vi "Fit Model to Plot Core.vi"(0 "Fit Plot Information":T6={"XY Graph Ref"=refnum, "Mouse Coordinates"={"X"=0.0, "Y"=0.0}, "Fit Model"=enum."Select a Fit Model...", "Plot Index"=-1}, 1 "LM Function & Gradient":refnum<vi>, 5 "Fit Settings":T3 {"Ramp Type" items=["Linear", "Logarithmic"]; "Fit Method" items=["Least Square", "Least Absolute Residual", "Bisquare"]}, 9 "Additional Data":variant, 11 "error in (no error)":errorcluster, 12 "Bin Location":T2, 13 "Send Graph to Notebook?":bool) -> (3 "Plot Name":string, 4 "Fitted Plot":cluster{"X Array":dbl[], "Y Array":dbl[]}, 6 "Fit Parameters Cluster":variant, 10 "Fit Parameters Uncertainties Cluster":variant, 14 "Fit Algorithm":T1, 15 "error out":errorcluster)   [LabVIEW 2019]
uses:
  Fit Plot Request Information.ctl
  <vilib>/Utility/miscctls.llb/LVPointDoubleTypeDef.ctl
  Fit Models.ctl
  Fit Settings.ctl
  <vilib>/Analysis/6fits.llb/Curve Fitting Criteria.ctl
  Ramp Type.ctl
  Histogram Bin Position.ctl
  Fit Algorithm.ctl
  LabVIEW Plot Interpolation.ctl
  Notebook.lvlib
  <vilib>/Analysis/NI_AALPro.lvlib
panel:
  in  "termination":cluster{"max iteration":i32, "tolerance":dbl}={"max iteration"=2000, "tolerance"=1e-09}
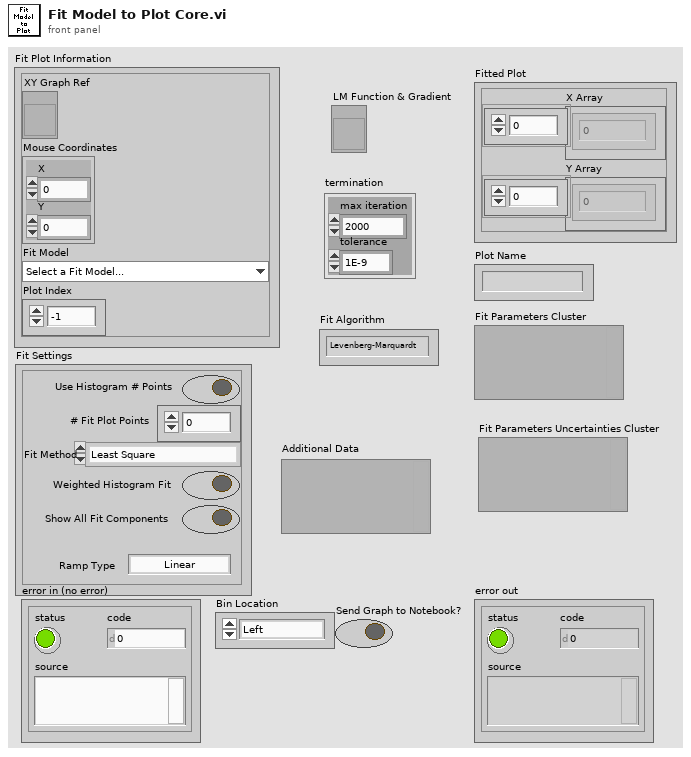
[diagram p1: front panel]
types:
  T1 = typedef "Fit Algorithm.ctl" = enum16{"Levenberg-Marquardt", "Trust-Region Dogleg"}
  T2 = typedef "Histogram Bin Position.ctl" = enum16{"Left", "Center", "Right"}
  T3 = typedef "Fit Settings.ctl" = cluster{"Use Histogram # Points":bool, "# Fit Plot Points":u32, "Fit Method":T4, "Weighted Histogram Fit":bool, "Show All Fit Components":bool, "Ramp Type":T5}
  T4 = typedef "NI_AALPro.lvlib/Curve Fitting Criteria.ctl" = u16
  T5 = typedef "Ramp Type.ctl" = u16
  T6 = typedef "Fit Plot Request Information.ctl" = cluster{"XY Graph Ref":refnum<vi>, "Mouse Coordinates":T7, "Fit Model":T8, "Plot Index":i32}
  T7 = typedef "LVPointDoubleTypeDef.ctl" = cluster{"X":dbl, "Y":dbl}
  T8 = typedef "Fit Models.ctl" = enum16{"Select a Fit Model...", "           Single Peak", "Gaussian", "Asymmetric Gaussian", "Lorentzian", "Asymmetric Lorentzian", "Gaussian/Lorentzian", "Lorentzian/Gaussian", "           Double Peak", "Two Gaussians", "Two Asymmetric Gaussians", "Two H-Connected Gaussians", "Two T-Connected Gaussians", "Two H-Connected Asymmetric Gaussians", "Two T-Connected Asymmetric Gaussians", "           Triple Peak", "Three Gaussians", "Three Asymmetric Gaussians", "              Decays", "Single Exponential", "Two Exponentials", "               ACF", "2D Gaussian ACF", "2D Gaussian + Blinking ACF", "2D Gaussian + Flow ACF", "3D Gaussian ACF", "3D Gaussian + Blinking ACF", "             Multiplot", "2D Gaussian ACF & 2D Gaussian + Flow ACF"}
  T9 = typedef "XY Graph Add-Ons.lvlib/XY Graph Refnum.ctl" = refnum<vi>
  T10 = cluster{"X Array out":dbl[], "Y Array out":dbl[], "Weights":dbl[]}
  T11 = cluster{"parameter minimum":dbl[], "parameter maximum":dbl[]}
  T12 = typedef "Fit Statistics.ctl" = cluster{"# iterations":i32, "number of function calls":i32, "chi2":dbl, "residue":dbl}
  T13 = cluster{"best fit parameters":dbl[], "best nonlinear fit":dbl[]}
  T14 = typedef "LabVIEW Plot Interpolation.ctl" = u8
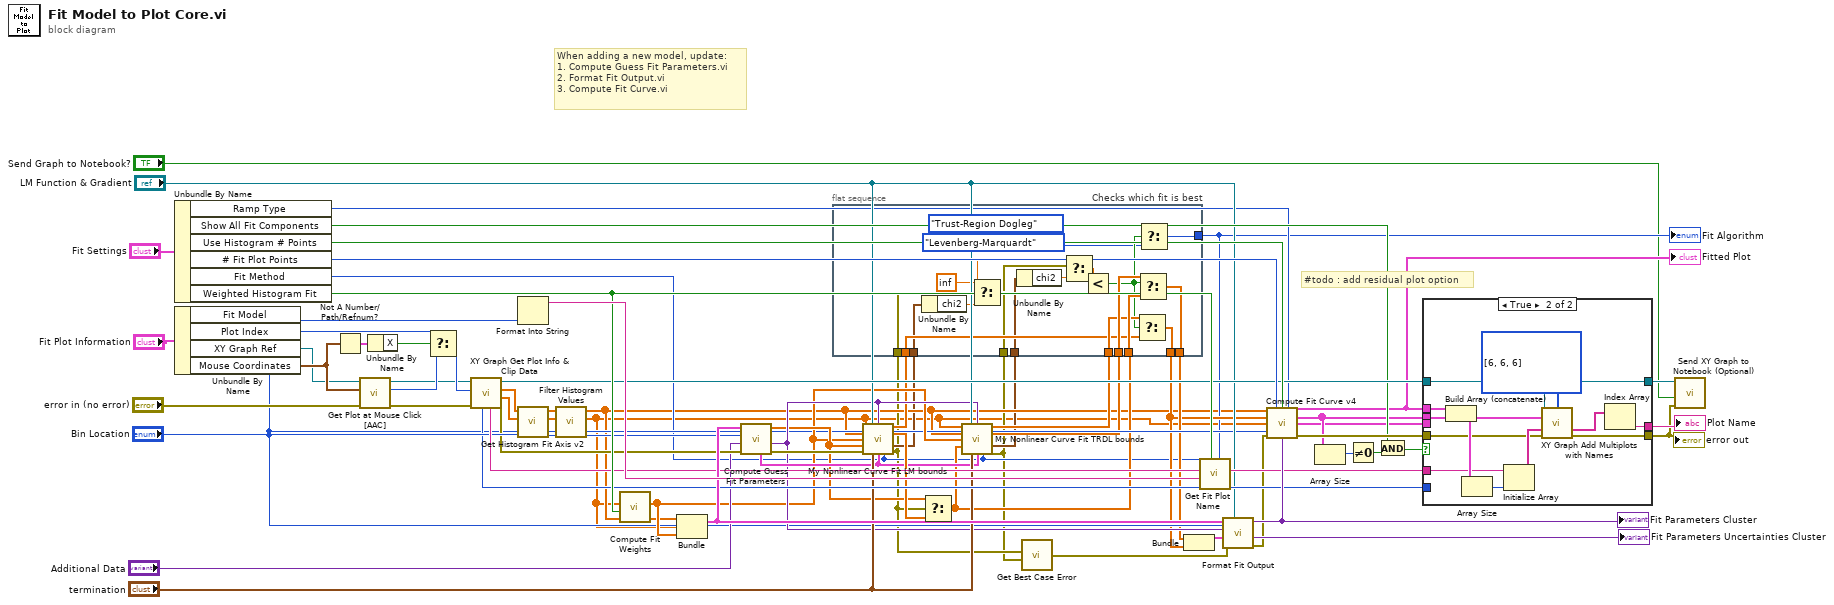
[diagram p0: block diagram]
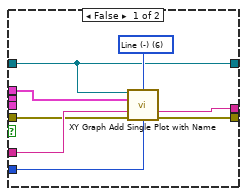
[diagram p2: hidden frame]
diagram:
  # "#todo : add residual plot option"
  # "When adding a new model, update:\n1. Compute Guess Fit Parameters.vi\n2. Format Fit Output.vi\n3. Compute Fit Curve.vi"
  n1 = Unbundle By Name("Fit Settings") -> ("Ramp Type"=w23:T5, "Show All Fit Components"=w35:bool, "Use Histogram # Points"=w61:bool, "# Fit Plot Points"=w62:u32, "Fit Method"=w12:T4, "Weighted Histogram Fit"=w64:bool)
  n2 = Unbundle By Name("Fit Plot Information") -> ("Fit Model"=w19:T8, "Plot Index"=w66:i32, "XY Graph Ref"=w67:refnum<vi>, "Mouse Coordinates"=w68:T7)
  n3 = Not A Number/Path/Refnum?(number/path/refnum=w68) -> (NaN/Path/Refnum?=w50:cluster{"X":bool, "Y":bool})
  n4 = call "Get Plot at Mouse Click [AAC].vi"("error in (no error)"="error in (no error)", "Mouse Click Coordinates"=w68, "XYGraph Ref"=w67) -> ("error out"=w44:errorcluster, "Plot at Coordinates"=w52:i32, "XYGraph Ref"=w42:T9)  [unwired: 2 in, 4 out]
  n5 = Unbundle By Name(w50) -> ("X"=w51:bool)
  n6 = Select(t=w66, s=w51, f=w52) -> (s? t:f=w53:i32)
  n7 = call "XY Graph Get Plot Info & Clip Data.vi"("error in (no error)"=w44, "Plot index"=w53, "XYGraph Ref in"=w42) -> ("error out"=w45:errorcluster, "Y Array"=w29:dbl[], "X Array"=w56:dbl[], "XYGraph Ref out"=w43:refnum<vi>, "Plot Name"=w54:string, "Plot Color"=w47:u32)  [unwired: 3 in]
  n8 = Format Into String(w19) -> (resulting string=w69:string)  [unwired: 3 in, 1 out]
  n9 = call "Get Histogram Fit Axis v2.vi"("Bin Location (Left)"="Bin Location", "Histogram Values"=w29, "Histogram Axis"=w56) -> ("Ordered Axis Histogram Values"=w9:dbl[], "Ordered Histogram Axis"=w10:dbl[])  [unwired: 3 in, 4 out]
  n10 = call "Filter Histogram Values.vi"("Y Array in"=w9, "X Array in"=w10) -> ("Y Array out"=w3:dbl[], "X Array out"=w8:dbl[])  [unwired: 7 in, 1 out]
  n11 = call "Compute Fit Weights.vi"("Use Weights? (F)"=w64, "Function Values"=w3) -> ("Weights"=w21:dbl[])  [unwired: 9 in]
  n12 = Bundle("X Array out"=w8, "Y Array out"=w3, "Weights"=w21) -> (w59:T10)  [unwired: 1 in]
  n13 = call "Compute Guess Fit Parameters.vi"("error in (no error)"=w45, "Additional Data"="Additional Data", "Fit Model"=w19, "Data in"=w59) -> ("error out"=w41:errorcluster, "Additional LM Data"=w24:variant, "Initial Fit Parameters"=w22:dbl[], "Parameter Bounds"=w26:T11)  [unwired: 4 in]
  n14 = flat-sequence "Checks which fit is best" {
    tunnel: w18 -> [w88]
    tunnel: w17 -> [w87]
    tunnel: [w86] -> w16
    tunnel: w15 -> [w85]
    tunnel: w14 -> [w84]
    tunnel: [w83] -> w13
    tunnel: [w79] -> w11
    tunnel: w6 -> [w78]
    tunnel: w7 -> [w77]
    tunnel: w5 -> [w75]
    tunnel: w4 -> [w71]
    frame #0 {
      w70 = inf ("t")
      n15 = Unbundle By Name(w77) -> ("chi2"=w76:dbl)
      n16 = Select(t=w70, s=w75, f=w76) -> (s? t:f=w74:dbl)
      n17 = Unbundle By Name(w78) -> ("chi2"=w73:dbl)
      n18 = Select(t=w70, s=w71, f=w73) -> (s? t:f=w72:dbl)
      n19 = Less?(x=w72, y=w74) -> (x < y?=w82:bool)
      n20 = Select(t=w85, s=w82, f=w84) -> (s? t:f=w83:dbl[])
      n21 = Select(t=w88, s=w82, f=w87) -> (s? t:f=w86:dbl[])
      n22 = Select(t=Fit_Algorithm."Trust-Region Dogleg" ("Fit Algorithm"), s=w82, f=Fit_Algorithm."Levenberg-Marquardt" ("Fit Algorithm")) -> (s? t:f=w79:T1)
    }
  }
  n23 = call "My Nonlinear Curve Fit LM bounds.vi"("Y"=w3, "f(x,a)"="LM Function & Gradient", "data"=w24, "X"=w8, "Weight"=w21, "initial parameters"=w22, "error in (no error)"=w41, "termination"="termination", "parameter bounds"=w26, "method"=w12) -> ("best nonlinear fit"=w14:dbl[], "best fit parameters"=w27:dbl[], "Fit Statistics"=w7:T12, "error out"=w5:errorcluster)  [unwired: 2 out]
  n24 = Select(t=w22, s=w5, f=w27) -> (s? t:f=w17:dbl[])
  n25 = call "My Nonlinear Curve Fit TRDL bounds.vi"("Y"=w3, "f(x,a)"="LM Function & Gradient", "data"=w24, "X"=w8, "Weight"=w21, "initial parameters"=w17, "termination"="termination", "parameter bounds"=w26, "method"=w12) -> ("best nonlinear fit"=w15:dbl[], "best fit parameters"=w18:dbl[], "Fit Statistics"=w6:T12, "error out"=w4:errorcluster)  [unwired: 1 in, 2 out]
  n26 = call "Get Best Case Error.vi"("error 2 in (no error)"=w4, "error 1 in (no error)"=w5) -> ("error out"=w20:errorcluster)  [unwired: 4 in]
  n27 = Bundle("best fit parameters"=w16, "best nonlinear fit"=w13) -> (w57:T13)  [unwired: 1 in]
  n28 = call "Get Fit Plot Name.vi"("Fit Algorithm"=w11, "Weighted Histogram Fit"=w64, "Fit Model"=w69, "Plot Name"=w54, "Fit Method"=w12) -> ("Fit Plot Name"=w55:string)  [unwired: 6 in]
  n29 = call "Format Fit Output.vi"("Fit Model"=w19, "f(x,a)"="LM Function & Gradient", "Error In"=w20, "Fit Results"=w57, "Additional Data"=w24, "Data in"=w59) -> ("Error Out"=w39:errorcluster, "Fit Parameters Uncertainties Cluster"=→"Fit Parameters Uncertainties Cluster":variant, "Fit Parameters Cluster"=w60:variant)  [unwired: 3 in]
  "Fit Parameters Cluster" <- w60
  n30 = call "Compute Fit Curve v4.vi"("X Array in"=w8, "# Points"=w62, "Use Same Number of Points as Histogram"=w61, "Best Fit in"=w13, "Y Array in"=w3, "Error In"=w39, "Fit Model"=w19, "Fit Parameters"=w60, "Ramp Type"=w23) -> ("Fitted Plot"=w33:cluster{"X Array":dbl[], "Y Array":dbl[]}, "Array of Component Plots"=w32:cluster{"X Array":dbl[], "Y Array":dbl[]}[], "Residual Plot"=w2:cluster{"X Array":dbl[], "Y Array":dbl[]}, "Error Out"=w46:errorcluster)  [unwired: 3 in]
  "Fitted Plot" <- w33
  n31 = Array Size(array=w32) -> (size(s)=w37:i32)
  n32 = Not Equal To 0?(x=w37) -> (x != 0?=w36:bool)
  n33 = And(x=w35, y=w36) -> (x .and. y?=w34:bool)
  n34 = case shown="True" w34 {
    tunnel: w55 -> [w96 w101]
    tunnel: [w94 w99] -> w30
    tunnel: [w93 w98] -> w48
    tunnel: w47 -> [w92 _]
    tunnel: w46 -> [w91 w100]
    tunnel: w43 -> [w89 w97]
    tunnel: w33 -> [w90 w103]
    tunnel: w32 -> [_ w102]
    tunnel: [w89 w97] -> w31
    tunnel: w2 -> [_ _]
    frame False {
      w95 = T14 6 items=["Point (.)", "Stepwise Right (--.)", "Stepwise Centered (-.-)", "Line + Point (\\. /)", "Stepwise Left (.--)", "Stepwise Vertical (|.|)", "Line (-)", "Use Previous Plot's Style"] ("Plot Interpolation (Previous Plot's Style)")
      n35 = call "XY Graph Add Single Plot with Name.vi"("XYGraph Ref in"=w89, "Plot Interpolation (Previous Plot's Style)"=w95, "Plot"=w90, "Plot Name (\"Plot\")"=w96, "error in (no error)"=w91, "Plot Color (Default)"=w92) -> ("Plot Name"=w93:string, "error out"=w94:errorcluster)  [unwired: 6 in, 2 out]
    }
    frame True {
      w104 = T14[] [6, 6, 6] items=["Point (.)", "Stepwise Right (--.)", "Stepwise Centered (-.-)", "Line + Point (\\. /)", "Stepwise Left (.--)", "Stepwise Vertical (|.|)", "Line (-)", "Use Previous Plot's Style"] ("Plots Interpolation (Previous Plot's Style)")
      n36 = Build Array (concatenate)(w103, w102) -> (w108:cluster{"X Array":dbl[], "Y Array":dbl[]}[])
      n37 = Array Size(array=w108) -> (size(s)=w107:i32)
      n38 = Initialize Array(w101, w107) -> (w106:string[])
      n39 = call "XY Graph Add Multiplots with Names.vi"("XYGraph in"=w97, "Plots Interpolation (Previous Plot's Style)"=w104, "Array of Plots"=w108, "Array of Plot Names (\"Plot\")"=w106, "error in (no error)"=w100) -> ("Added Plot Names"=w105:string[], "error out"=w99:errorcluster)  [unwired: 6 in, 3 out]
      n40 = Index Array(array=w105) -> (element=w98:string)  [unwired: 1 in]
    }
  }
  "error out" <- w30
  "Plot Name" <- w48
  n41 = call "Send XY Graph to Notebook (Optional).vi"("error in (no error)"=w30, "Send Graph to Notebook?"="Send Graph to Notebook?", "XYGraph in"=w31) -> ()  [unwired: 8 in, 1 out]
  "Fit Algorithm" <- w11
